vi "CalculateZoom(SubVI).vi"(10 "Compress the picture?":bool, 11 "VI in":refnum<vi>) -> (3 "Zoom":dbl)   [LabVIEW 2018]
panel:
  out "Error Out":errorcluster
  in  "Error In":errorcluster
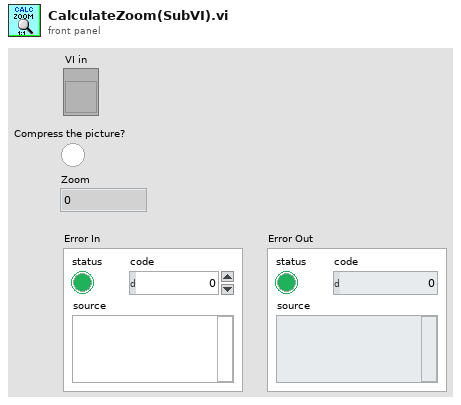
[diagram p1: front panel]
types:
  T1 = typedef "LVRectTypeDef.ctl" = cluster{"Left":i16, "Top":i16, "Right":i16, "Bottom":i16}
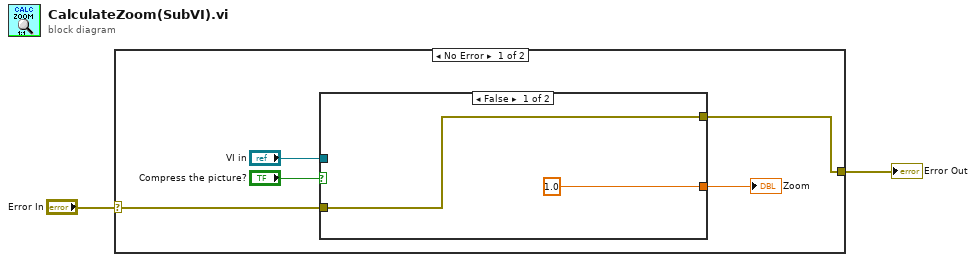
[diagram p0: block diagram]
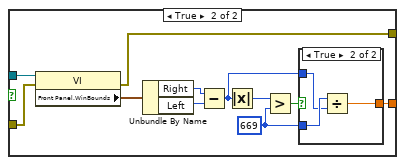
[diagram p2: hidden frame]
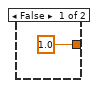
[diagram p3: hidden frame]
diagram:
  n1 = case shown="No Error" "Error In" {
    selector: "Error In" -> [w4 w25]
    tunnel: [w3 w25] -> w1
    frame No Error {
      n2 = case shown="False" "Compress the picture?" {
        tunnel: "VI in" -> [_ w19]
        tunnel: [1.0 w12] -> w5
        tunnel: w4 -> [w8 w11]
        tunnel: [w8 w10] -> w3
        frame False {
        }
        frame True {
          w14 = i16 669 ("y")
          n3 = property class="VI"(reference=w19, error in=w11) -> (error out=w10:errorcluster, "Front Panel.WinBounds"=w20:T1)  [unwired: 1 out]
          n4 = Unbundle By Name(w20) -> ("Right"=w18:i16, "Left"=w17:i16)
          n5 = Subtract(x=w18, y=w17) -> (x-y=w13:i16)
          n6 = Absolute Value(x=w13) -> (abs(x)=w16:i16)
          n7 = Greater?(x=w16, y=w14) -> (0:w15:bool)
          n8 = case shown="True" w15 {
            tunnel: w14 -> [_ w24]
            tunnel: w13 -> [_ w23]
            tunnel: [1.0 w22] -> w12
            frame False {
            }
            frame True {
              n9 = Divide(x=w24, y=w23) -> (x/y=w22:dbl)
            }
          }
        }
      }
      "Zoom" <- w5
    }
    frame Error {
    }
  }
  "Error Out" <- w1
